vi "Initialize Scope.vi"(8 "error in":errorcluster, 10 "Scope Settings":T1={"Scope Config File Path"=path "", "Reference Position"=50.0, "Number of Records"=0} {"Reference Position" format="%#_g%"}, 11 "Scope Resource":refnum<k15>) -> (0 "error out":errorcluster, 3 "Scope Resource":refnum<k15>)   [LabVIEW 2025]
uses:
  <instrlib>/niScope/Configure/niScope Import Attribute Configuration File.vi
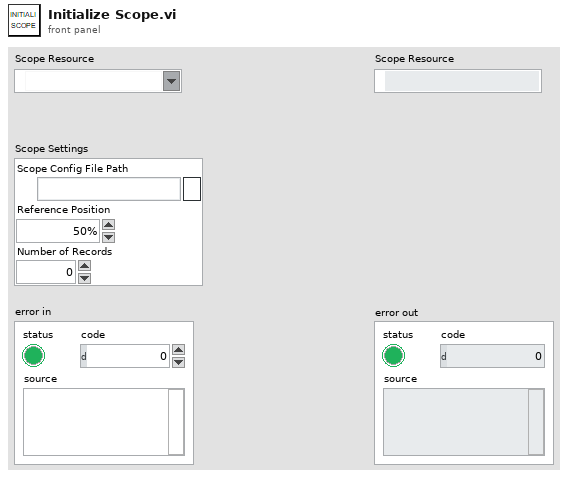
[diagram p1: front panel]
types:
  T1 = cluster{"Scope Config File Path":path, "Reference Position":dbl, "Number of Records":i32}
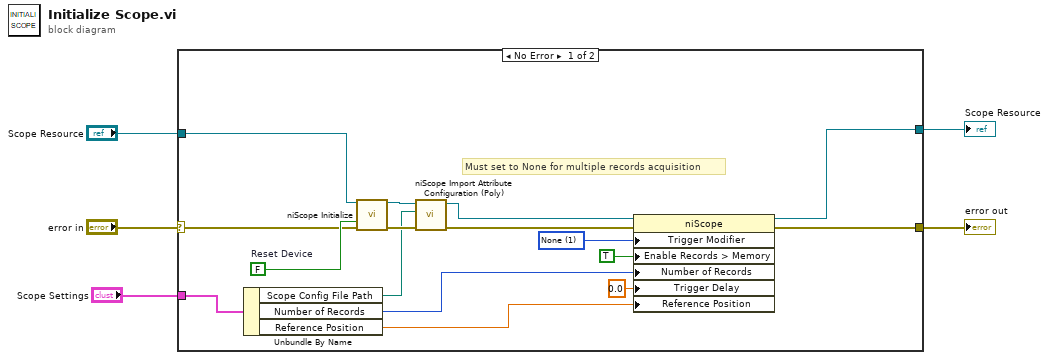
[diagram p0: block diagram]
diagram:
  n1 = case shown="No Error" "error in" {
    selector: "error in" -> [w13 w23]
    tunnel: [w21 w23] -> w5
    tunnel: [w20 w22] -> w4
    tunnel: "Scope Resource" -> [w15 w22]
    tunnel: "Scope Settings" -> [w12 _]
    frame No Error {
      w8 = 1 items=["None"=1, "Auto Trigger"=2] ("Triggering:Trigger Modifier")
      w14 = FALSE  # Reset Device
      # "Must set to None for multiple records acquisition"
      n2 = Unbundle By Name(w12) -> ("Scope Config File Path"=w11:path, "Number of Records"=w10:i32, "Reference Position"=w7:dbl)
      n3 = call <instrlib>:"niScope Initialize.vi"("resource name"=w15, "reset device"=w14, "error in"=w13) -> ("instrument handle"=w19:refnum<k15>, "error out"=w18:errorcluster)  [unwired: 11 in]
      n4 = call-poly <instrlib>:"niScope Import Attribute Configuration (Poly).vi"("error in"=w18, "file path"=w11, "instrument handle"=w19) -> ("error out"=w16:errorcluster, "instrument handle out"=w17:refnum<k15>)  [unwired: 7 in]
      n5 = property class="niScope"(reference=w17, error in=w16, "Trigger Modifier"=w8, "Enable Records > Memory"=TRUE ("Horizontal:Enable Records > Memory"), "Number of Records"=w10, "Trigger Delay"=0.0 ("Triggering:Trigger Delay"), "Reference Position"=w7) -> (reference out=w20:refnum<k15>, error out=w21:errorcluster)
    }
    frame Error {
    }
  }
  "error out" <- w5
  "Scope Resource" <- w4
